vi "Test Parser.vi"() -> ()   [LabVIEW 2014]
uses:
  C:/Files/Custom VeriStand Development/DET-SPI-Tool/Source/System Explorer/Runtime Menu Items/SLSC Deserializer.dll
  Source/System Explorer/Runtime Menu Items/SLSC Deserializer.dll
panel:
  in  "Write Path":path
  out "Array 2":bool[](array[boolean])
  out "Array":string[](array[string])
  in  "Path":path
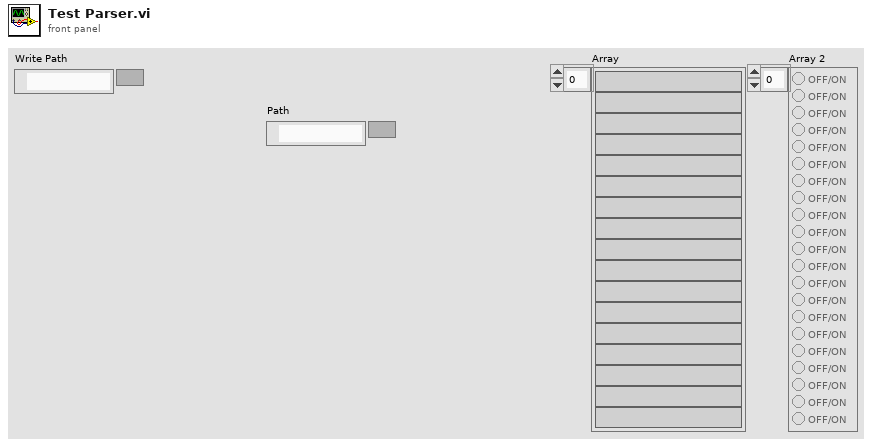
[diagram p1: front panel]
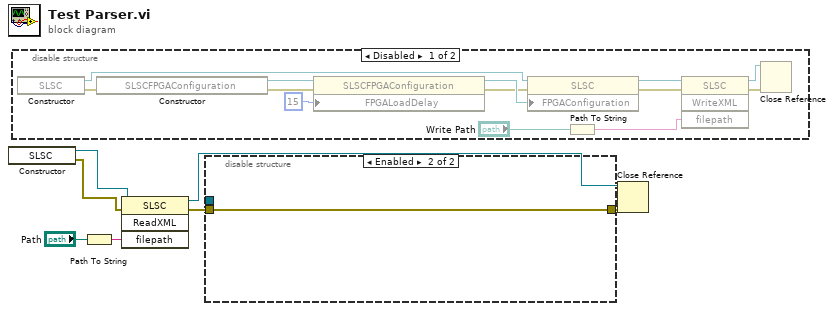
[diagram p0: block diagram]
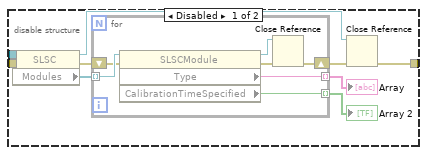
[diagram p3: hidden frame]
diagram:
  n1 = constructor class="SLSC"() -> (reference out=w1:refnum<k24>, error out=w2:errorcluster)  [unwired: 3 in, 1 out]
  n2 = disable-structure shown="Disabled" {
    frame Disabled {
      n3 = constructor class="SLSC"() -> (reference out=w11:refnum<k24>, error out=w10:errorcluster)  [unwired: 3 in, 1 out]
      n4 = constructor class="SLSCFPGAConfiguration"(error in=w10) -> (reference out=w15:refnum<k24>, error out=w14:errorcluster)  [unwired: 2 in, 1 out]
      n5 = property class="SLSCFPGAConfiguration"(reference=w15, error in=w14, "FPGALoadDelay"=i8 15) -> (reference out=w13:refnum<k24>, error out=w12:errorcluster)
      n6 = property class="SLSC"(reference=w11, error in=w12, "FPGAConfiguration"=w13) -> (reference out=w8:refnum<k24>, error out=w9:errorcluster)
      n7 = Path To String(path="Write Path") -> (string=w17:string)
      n8 = invoke class="SLSC" method="WriteXML"(reference=w8, error in=w9, "filepath"=w17) -> (reference out=w18:refnum<k24>, error out=w19:errorcluster)  [unwired: 1 in, 2 out]
      n9 = Close Reference(reference=w18, error in (no error)=w19) -> ()  [unwired: 1 out]
    }
    frame Enabled {
    }
  }
  n10 = Path To String(path="Path") -> (string=w3:string)
  n11 = invoke class="SLSC" method="ReadXML"(reference=w1, error in=w2, "filepath"=w3) -> (reference out=w4:refnum<k24>, error out=w5:errorcluster)  [unwired: 1 in, 2 out]
  n12 = disable-structure shown="Enabled" {
    disable-tunnel: _ -> [w29 _]
    disable-tunnel: w5 -> [w28 w37]
    disable-tunnel: [w22 w37] -> w6
    frame Disabled {
      n13 = property class="SLSC"(reference=w29, error in=w28) -> (reference out=w23:refnum<k24>, error out=w26:errorcluster, "Modules"=w27:refnum<k24>[])
      n14 = for {
        tunnel: w27 -> [w36] mode=indexing
        shift-right: [w33] -> w24
        shift-left: w26 -> [w35]
        tunnel: [w34] -> w25 mode=indexing
        tunnel: [w30] -> w21 mode=indexing
        n15 = property class="SLSCModule"(reference=w36, error in=w35) -> (reference out=w31:refnum<k24>, error out=w32:errorcluster, "Type"=w34:string, "CalibrationTimeSpecified"=w30:bool)
        n16 = Close Reference(reference=w31, error in (no error)=w32) -> (error out=w33:errorcluster)
      }
      "Array" <- w25
      "Array 2" <- w21
      n17 = Close Reference(reference=w23, error in (no error)=w24) -> (error out=w22:errorcluster)
    }
    frame Enabled {
    }
  }
  n18 = Close Reference(reference=w4, error in (no error)=w6) -> ()  [unwired: 1 out]
